vi "Main.vi"(8 "error in":errorcluster, 11 "Server Client in":refnum<class "Server Client.lvclass">) -> (0 "error out":errorcluster, 3 "Server Client out":refnum<class "Server Client.lvclass">)   [LabVIEW 2020, in "Server Client.lvclass"]
doc: "The Queued Message Handler of a Worker."
uses:
  Server Client.lvclass
  <vilib>/addons/_Workers/Library/Classes/EHL/EHL.lvclass
  <vilib>/addons/_Workers/Library/Classes/Worker/Worker.lvclass
  <vilib>/addons/_Workers/Library/Classes/Error Handler/Error Handler.lvclass
  Initialization Data.ctl
  Listener/Listener.lvclass
  <vilib>/addons/_Workers/Library/Classes/Message/Message.lvclass
  <vilib>/addons/_Workers/Library/Classes/Message/Enqueue Message to Queue.vi
  Network End Point/Network End Point.lvclass
  Network End Point/Initialization Data.ctl
  <vilib>/addons/_Workers/Library/Classes/Message Queue/Message Queue.lvclass
  <vilib>/addons/_Workers/Library/Classes/Message/Enqueue Message to Self.vi
  C:/Program Files (x86)/National Instruments/LabVIEW 2020/vi.lib/addons/_Workers/Library/Classes/Worker User/Worker User.lvclass
  C:/Program Files (x86)/National Instruments/LabVIEW 2020/vi.lib/addons/_Workers/Library/Classes/Worker/Worker.lvclass
  C:/Program Files (x86)/National Instruments/LabVIEW 2020/vi.lib/addons/_Workers/Library/Classes/Workers Object/Workers Object.lvclass
  C:/Users/TestAdmin/git/TCP-Workers/Workers/Server Client/Server Client.lvclass
  C:/Users/TestAdmin/git/TCP-Workers/Workers/Listener/Listener.lvclass
  C:/Program Files (x86)/National Instruments/LabVIEW 2020/vi.lib/addons/_Workers/Library/Classes/Message Queue/Message Queue.lvclass
  C:/Users/TestAdmin/git/TCP-Workers/Workers/Network End Point/Network End Point.lvclass
panel:
  in  "Connect to":string
  in  "Open":bool
  in  "Open Listener":bool
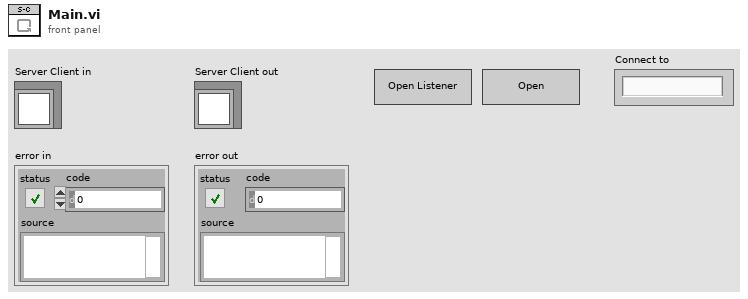
[diagram p1: front panel]
types:
  T1 = typedef "Server Client.lvclass/Initialization Data.ctl" = cluster{"String":string, "port":u16}
  T2 = typedef "Network End Point.lvclass/Initialization Data.ctl" = cluster{"String":string, "Client":string, "connection ID":refnum<k5>, "Caller":refnum<class "Message Queue.lvclass">}
  T3 = typedef "Workers.lvlib/Case Label.ctl" = string
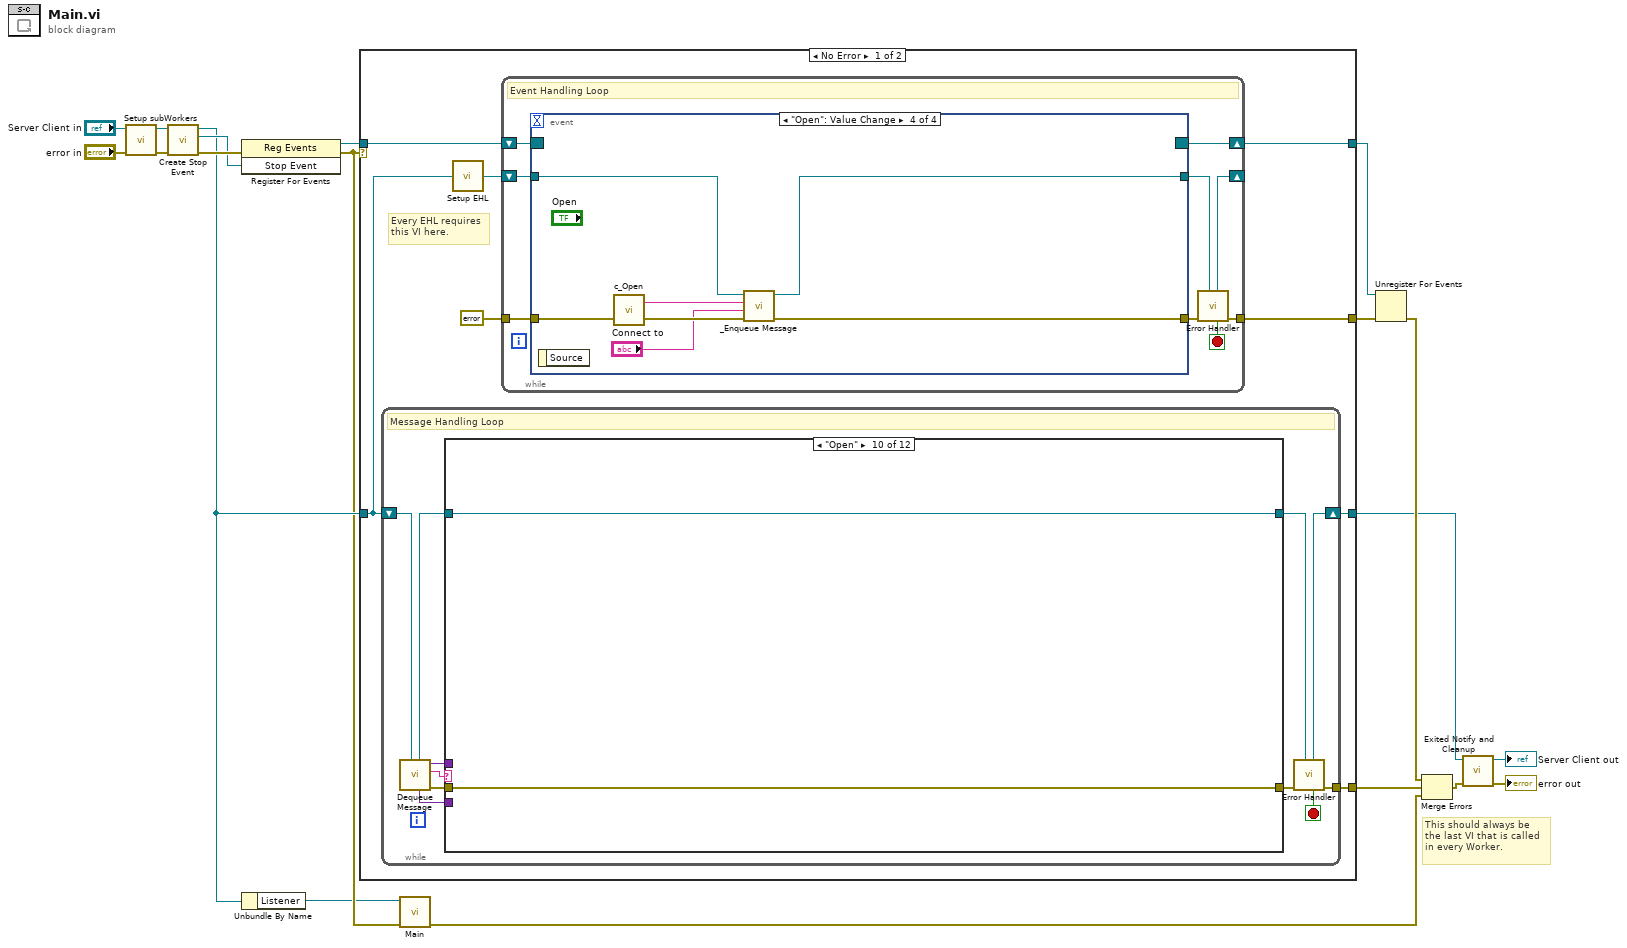
[diagram p0: block diagram]
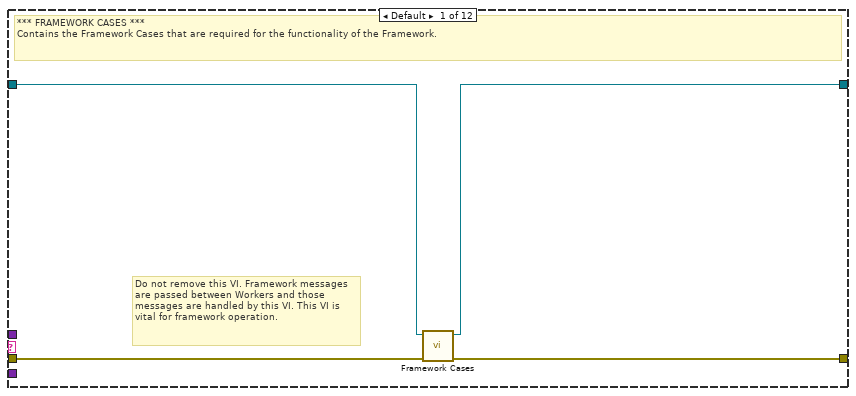
[diagram p2: hidden frame]
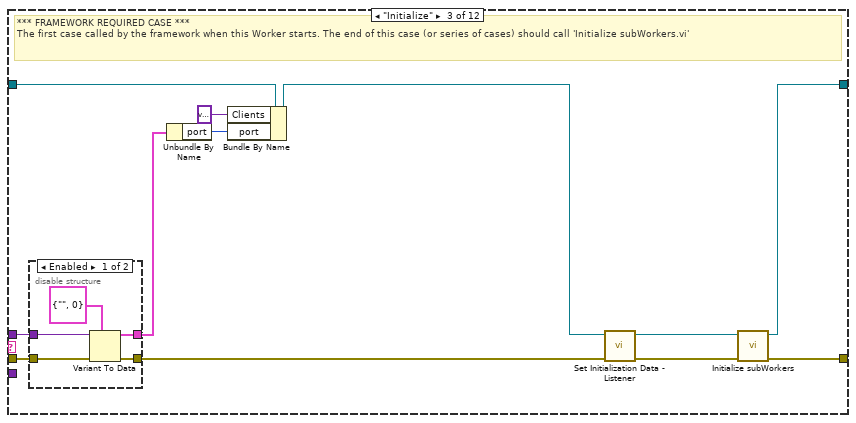
[diagram p4: hidden frame]
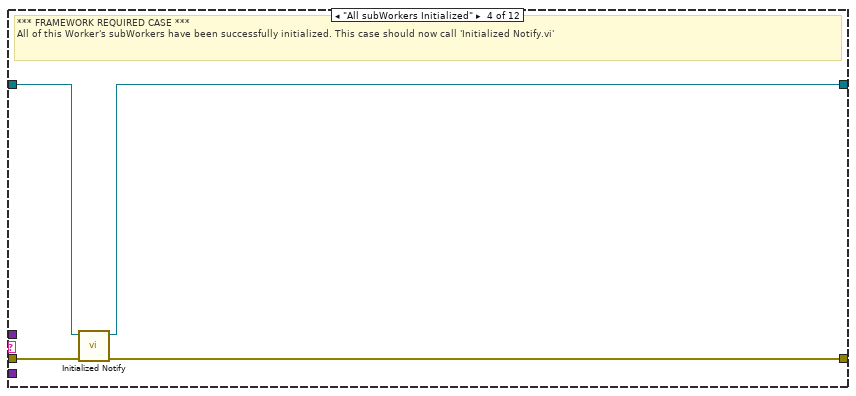
[diagram p6: hidden frame]
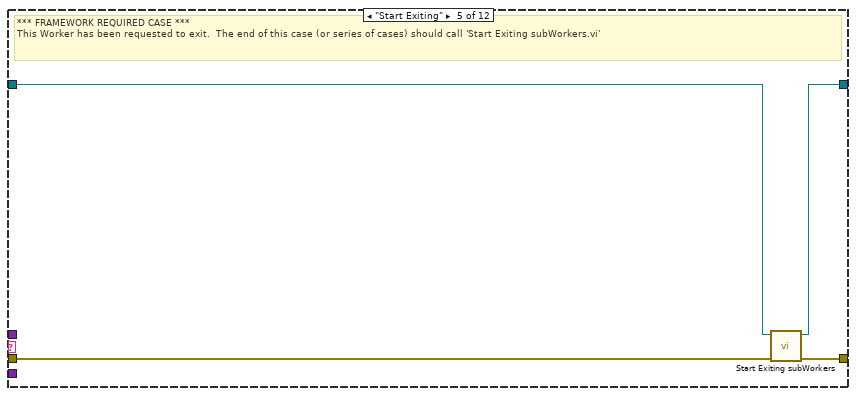
[diagram p7: hidden frame]
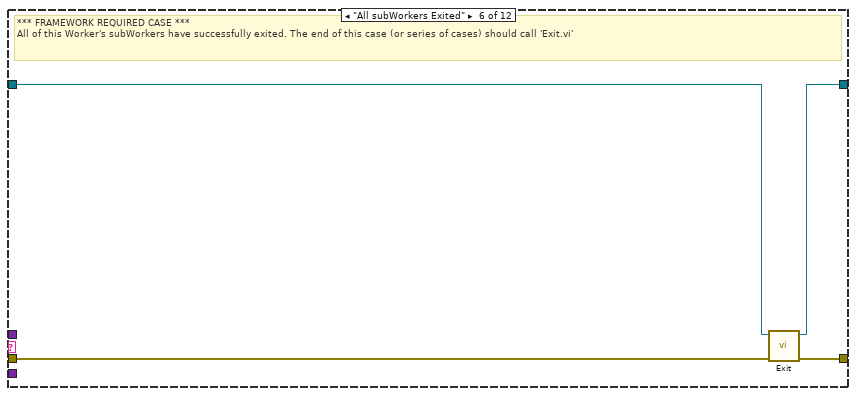
[diagram p8: hidden frame]
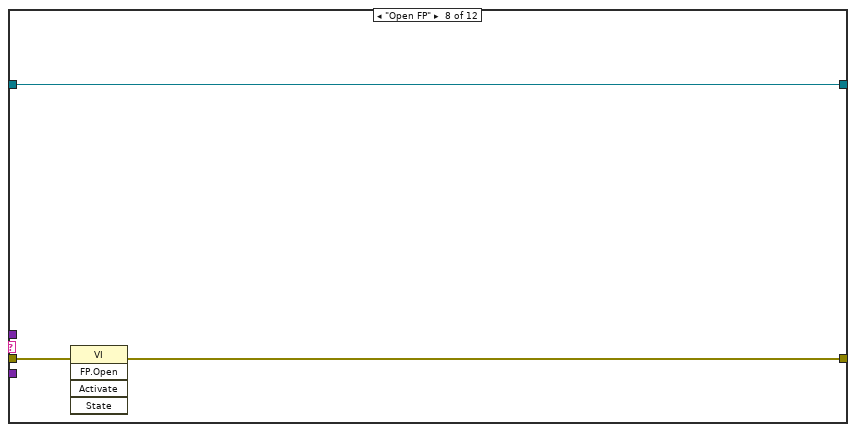
[diagram p10: hidden frame]
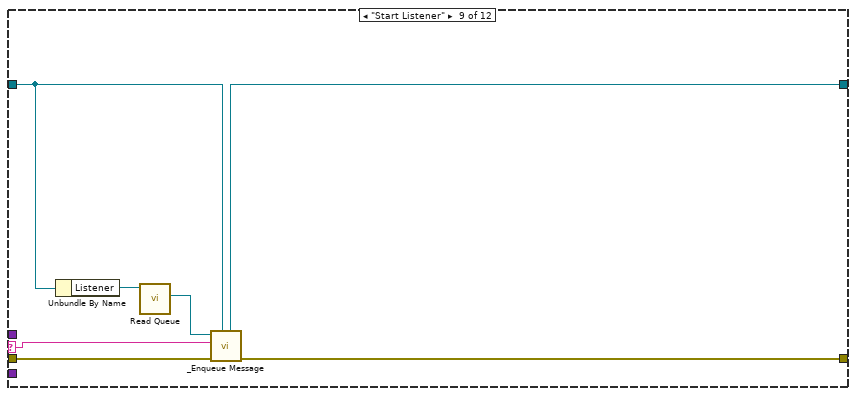
[diagram p11: hidden frame]
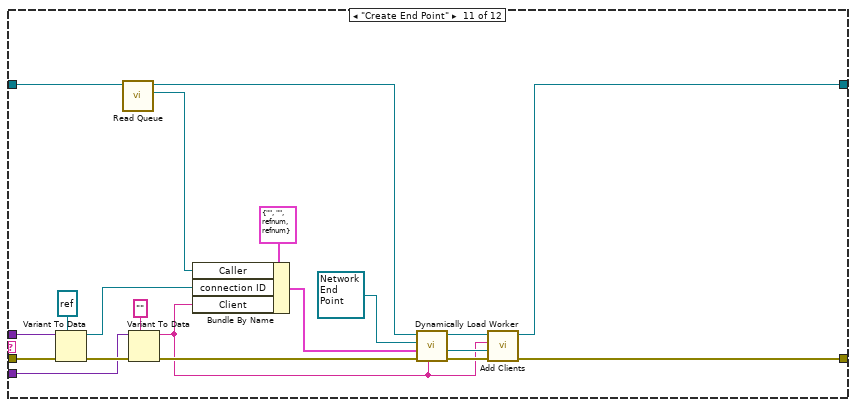
[diagram p12: hidden frame]
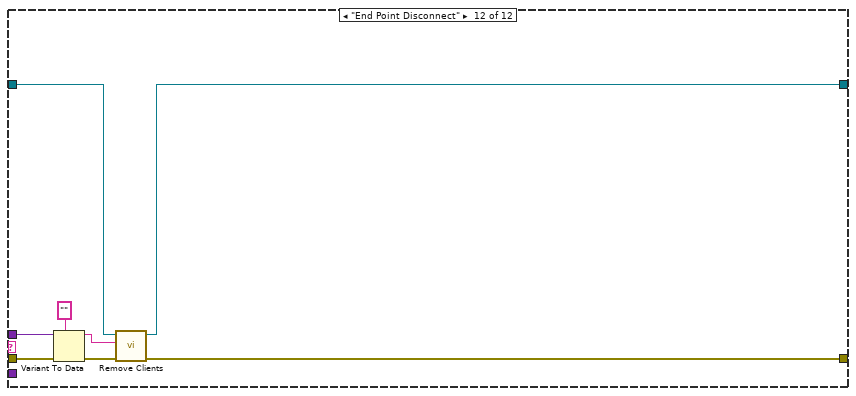
[diagram p13: hidden frame]
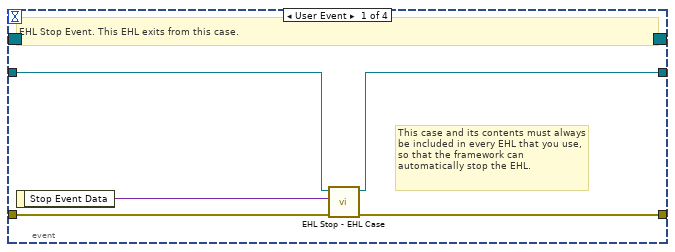
[diagram p14: hidden frame]
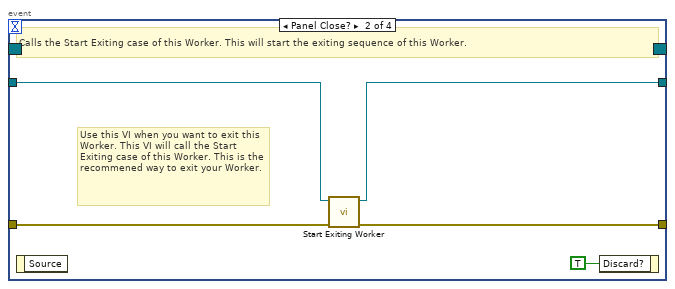
[diagram p15: hidden frame]
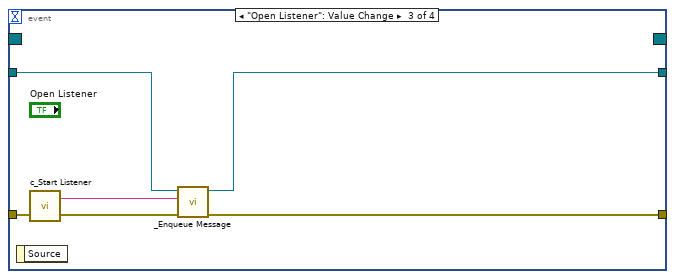
[diagram p16: hidden frame]
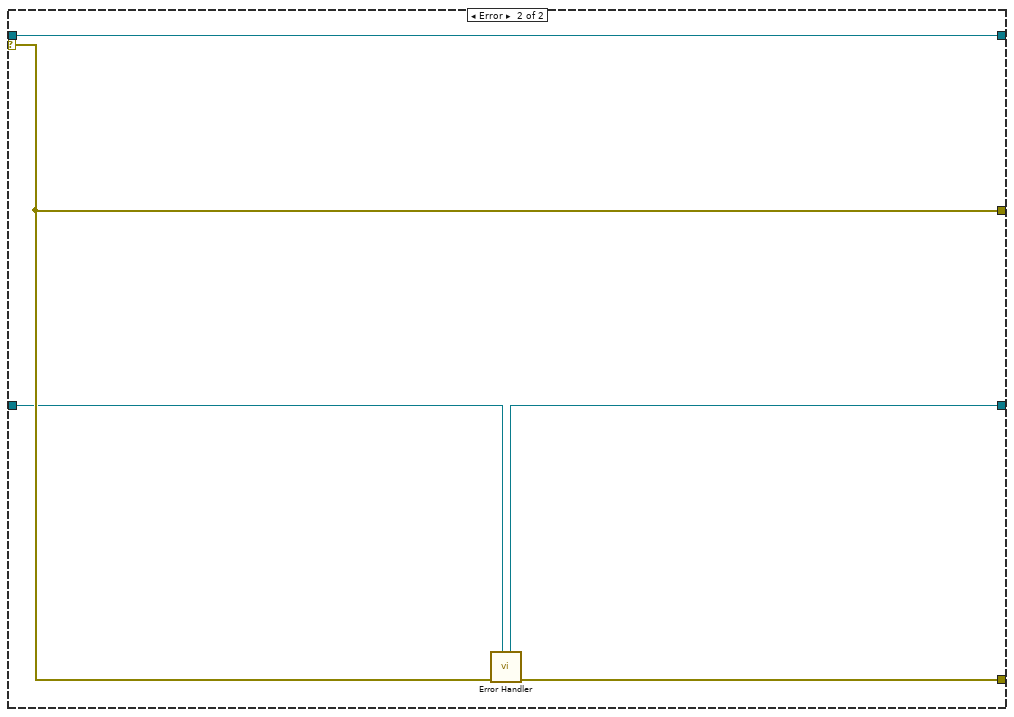
[diagram p17: hidden frame]
diagram:
  # "This should always be the last VI that is called in every Worker."
  n1 = call "Setup subWorkers.vi"("error in"="error in", "Server Client in"="Server Client in") -> ("error out"=w5:errorcluster, "Server Client out"=w3:refnum<class "Server Client.lvclass">)  [unwired: 8 in]
  n2 = call <vilib>:"Create Stop Event.vi"("error in"=w5, "Worker"=w3) -> ("error out"=w14:errorcluster, "Stop Event"=w11:refnum<user-event>, "Worker out"=w8:refnum<class "Server Client.lvclass">)  [unwired: 7 in]
  n3 = register-events(error in=w14, w11) -> (reference out=w13:refnum<event-registration>, error out=w6:errorcluster)  [unwired: 1 in]
  n4 = Unbundle By Name(w8) -> ("Listener"=w2:refnum<class "Listener.lvclass">)
  n5 = case shown="No Error" w6 {
    tunnel: w8 -> [w22 w148]
    tunnel: [w20 w149] -> w12
    tunnel: w13 -> [w27 w150]
    tunnel: [w24 w151] -> w18
    tunnel: [w26 w150] -> w17
    tunnel: [w21 w147] -> w15
    selector: w6 -> [_ w151]
    frame No Error {
      # "Every EHL requires\nthis VI here."
      n6 = while {
        shift-right: [w36] -> w21
        shift-left: w22 -> [w38]
        tunnel: [w37] -> w20
        stop <- w29 stop-if-true
        # "Message Handling Loop"
        n7 = call <vilib>:"Dequeue Message.vi"("Worker"=w38) -> ("error out"=w35:errorcluster, "Case out"=w30:string, "Data out"=w31:variant, "Auxiliary out"=w28:variant, "Worker out"=w33:refnum<class "Server Client.lvclass">)  [unwired: 6 in]
        n8 = case "WORKERS MHL Case Structure (DO NOT CHANGE LABEL NAME)" shown="\"Open\"" w30 {
          selector: w30 -> [_ _ _ _ _ _ _ _ w83 _ _ _]
          tunnel: w35 -> [w42 w43 w54 w66 w67 w74 w75 w79 w86 w87 w108 w116]
          tunnel: [w41 w43 w56 w65 w70 w73 w75 w77 w80 w87 w91 w112] -> w34
          tunnel: w33 -> [w40 w44 w52 w63 w68 w71 w76 w78 w82 w88 w96 w110]
          tunnel: [w39 w44 w55 w64 w69 w72 w76 w78 w81 w88 w93 w109] -> w32
          tunnel: w31 -> [_ _ w53 _ _ _ _ _ _ _ w107 w114]
          tunnel: w28 -> [_ _ _ _ _ _ _ _ _ _ w105 _]
          frame Default {
            # "Do not remove this VI. Framework messages are passed between Workers and those messages are handled by this VI. This VI is vital for framework operation."
            # "*** FRAMEWORK CASES ***\nContains the Framework Cases that are required for the functionality of the Framework."
            n9 = call <vilib>:"Framework Cases.vi"("error in"=w42, "Worker"=w40) -> ("error out"=w41:errorcluster, "Worker out"=w39:refnum<class "Server Client.lvclass">)  [unwired: 8 in]
          }
          frame "------ FRAMEWORK REQUIRED CASES ------" {
            # "Start of Framework Required Cases"
          }
          frame "Initialize" {
            # "*** FRAMEWORK REQUIRED CASE ***\nThe first case called by the framework when this Worker starts. The end of this case (or series of cases) should call 'Initialize subWorkers.vi'"
            n10 = disable-structure shown="Enabled" {
              disable-tunnel: w54 -> [w61 w62]
              disable-tunnel: [w60 w62] -> w49
              disable-tunnel: w53 -> [w59 _]
              disable-tunnel: [w57 _] -> w51
              frame Enabled {
                n11 = Variant To Data(error in=w61, type=T1 {"String"="", "port"=0} ("Initialization Data"), Variant=w59) -> (data=w57:T1, error out=w60:errorcluster)
              }
              frame Disabled {
              }
            }
            n12 = Unbundle By Name(w51) -> ("port"=w50:u16)
            n13 = Bundle By Name(cluster=w52, "Clients"=variant, "port"=w50) -> (w47:refnum<class "Server Client.lvclass">)
            n14 = call "Set Initialization Data - Listener.vi"("error in"=w49, "Server Client in"=w47) -> ("error out"=w48:errorcluster, "Server Client out"=w46:refnum<class "Server Client.lvclass">)  [unwired: 8 in]
            n15 = call <vilib>:"Initialize subWorkers.vi"("error in"=w48, "Worker"=w46) -> ("error out"=w56:errorcluster, "dup Worker out"=w55:refnum<class "Server Client.lvclass">)  [unwired: 8 in]
          }
          frame "All subWorkers Initialized" {
            # "*** FRAMEWORK REQUIRED CASE ***\nAll of this Worker's subWorkers have been successfully initialized. This case should now call 'Initialized Notify.vi'"
            n16 = call <vilib>:"Initialized Notify.vi"("error in"=w66, "Worker"=w63) -> ("error out"=w65:errorcluster, "dup Worker out"=w64:refnum<class "Server Client.lvclass">)  [unwired: 8 in]
          }
          frame "Start Exiting" {
            # "*** FRAMEWORK REQUIRED CASE ***\nThis Worker has been requested to exit.  The end of this case (or series of cases) should call 'Start Exiting subWorkers.vi'"
            n17 = call <vilib>:"Start Exiting subWorkers.vi"("error_in"=w67, "Worker"=w68) -> ("error out"=w70:errorcluster, "dup Worker out"=w69:refnum<class "Server Client.lvclass">)  [unwired: 8 in]
          }
          frame "All subWorkers Exited" {
            # "*** FRAMEWORK REQUIRED CASE ***\nAll of this Worker's subWorkers have successfully exited. The end of this case (or series of cases) should call 'Exit.vi'"
            n18 = call <vilib>:"Exit.vi"("error_in"=w74, "Worker"=w71) -> ("error out"=w73:errorcluster, "dup Worker out"=w72:refnum<class "Server Client.lvclass">)  [unwired: 8 in]
          }
          frame "-----------------------------------------------" {
            # "End of Framework Required Cases"
          }
          frame "Open FP" {
            n19 = invoke class="VI" method="FP.Open"(error in=w79) -> (error out=w77:errorcluster)  [unwired: 4 in, 4 out]
          }
          frame "Start Listener" {
            n20 = Unbundle By Name(w82) -> ("Listener"=w85:refnum<class "Listener.lvclass">)
            n21 = call <vilib>:"Read Queue.vi"("Worker"=w85) -> ("Message Queue out"=w84:refnum<class "Message Queue.lvclass">)  [unwired: 9 in, 1 out]
            n22 = call-poly <vilib>:"_Enqueue Message.vi"("Worker"=w82, "error in"=w86, "Case Label"=w83, "Message Queue"=w84) -> ("error out"=w80:errorcluster, "dup Worker out"=w81:refnum<class "Server Client.lvclass">)  [unwired: 5 in, 1 out]
          }
          frame "Open" {
          }
          frame "Create End Point" {
            n23 = Variant To Data(error in=w108, type=refnum<k5> refnum ("connection ID"), Variant=w107) -> (data=w97:refnum<k5>, error out=w106:errorcluster)
            n24 = call <vilib>:"Read Queue.vi"("Worker"=w96) -> ("Message Queue out"=w94:refnum<class "Message Queue.lvclass">, "dup Worker out"=w95:refnum<class "Server Client.lvclass">)  [unwired: 9 in]
            n25 = Variant To Data(error in=w106, type="", Variant=w105) -> (data=w89:string, error out=w102:errorcluster)
            n26 = Bundle By Name(cluster=T2 {"String"="", "Client"="", "connection ID"=refnum, "Caller"=refnum} ("Initialization Data"), "Caller"=w94, "connection ID"=w97, "Client"=w89) -> (w98:T2)
            n27 = call <vilib>:"Dynamically Load Worker.vi"("Worker Alias"=w89, "error in"=w102, "Initialization Data"=w98, "Worker to Dynamically Load"=refnum<class "Network End Point.lvclass"> refnum ("Network End Point.lvclass"), "Worker"=w95) -> ("error out"=w92:errorcluster, "Message Queue out"=w90:refnum<class "Message Queue.lvclass">, "dup Worker out"=w101:refnum<class "Server Client.lvclass">)  [unwired: 3 in, 1 out]
            n28 = call "Add Clients.vi"("error in (no error)"=w92, "End Point Queue"=w90, "Client"=w89, "Server Client in"=w101) -> ("error out"=w91:errorcluster, "Server Client out"=w93:refnum<class "Server Client.lvclass">)  [unwired: 6 in]
          }
          frame "End Point Disconnect" {
            n29 = Variant To Data(error in=w116, type="", Variant=w114) -> (data=w111:string, error out=w115:errorcluster)
            n30 = call "Remove Clients.vi"("error in (no error)"=w115, "Client"=w111, "Server Client in"=w110) -> ("error out"=w112:errorcluster, "Server Client out"=w109:refnum<class "Server Client.lvclass">)  [unwired: 7 in]
          }
        }
        n31 = call <vilib>:"Error Handler.vi"("Worker"=w32, "error_in"=w34) -> ("error out"=w37:errorcluster, "Stop Loop"=w29:bool, "Worker out"=w36:refnum<class "Server Client.lvclass">)  [unwired: 7 in]
      }
      n32 = call <vilib>:"Setup EHL.vi"("Worker"=w22) -> ("Worker out"=w23:refnum<class "Server Client.lvclass">)  [unwired: 14 in]
      n33 = while "Event Handling Loop" {
        shift-right: [w125] -> w26
        shift-left: w27 -> [w124]
        tunnel: [w120] -> w24
        tunnel: errorcluster {"status"=FALSE, "code"=0, "source"=""} ("error constant") -> [w122]
        shift-right: [w118] -> _
        shift-left: w23 -> [w123]
        stop <- w117 stop-if-true
        # "Event Handling Loop"
        n34 = event shown="[3] \"Open\": Value Change" {
          selector: w124 -> [_ _ _ _]
          dyn-events: [_ _ _ _] -> w125
          timeout: _ -> [_ _ _ _]
          tunnel: [w129 w134 w139 w145] -> w121
          tunnel: w122 -> [w130 w133 w140 w146]
          tunnel: w123 -> [w128 w132 w138 w144]
          tunnel: [w127 w131 w137 w143] -> w119
          event User Event {
            # "This case and its contents must always be included in every EHL that you use, so that the framework can automatically stop the EHL."
            # "EHL Stop Event. This EHL exits from this case."
            n35 = event-data() -> ("Stop Event Data"=w126:variant)  [unwired: 1 in]
            n36 = call <vilib>:"EHL Stop - EHL Case.vi"("error in"=w130, "Stop Event Data"=w126, "Worker"=w128) -> ("error out"=w129:errorcluster, "Worker out"=w127:refnum<class "Server Client.lvclass">)  [unwired: 7 in]
          }
          event Panel Close? {
            # "Use this VI when you want to exit this Worker. This VI will call the Start Exiting case of this Worker. This is the recommened way to exit your Worker."
            # "Calls the Start Exiting case of this Worker. This will start the exiting sequence of this Worker."
            n37 = event-data() -> ()  [unwired: 1 in, 1 out]
            n38 = call <vilib>:"Start Exiting Worker.vi"("error in"=w133, "Worker"=w132) -> ("error out"=w134:errorcluster, "dup Worker out"=w131:refnum<class "Server Client.lvclass">)  [unwired: 8 in]
            n39 = event-data ("Event Filter Node")("Discard?"=TRUE) -> ()  [unwired: 1 in, 1 out]
          }
          event "Open Listener": Value Change {
            n40 = event-data() -> ()  [unwired: 1 in, 1 out]
            n41 = call "c_Start Listener.vi"() -> ("Case Label"=w136:T3)  [unwired: 1 in]
            n42 = call-poly <vilib>:"_Enqueue Message.vi"("error in"=w140, "Case Label"=w136, "Worker"=w138) -> ("error out"=w139:errorcluster, "dup Worker out"=w137:refnum<class "Server Client.lvclass">)  [unwired: 7 in]
          }
          event "Open": Value Change {
            n43 = event-data() -> ()  [unwired: 1 in, 1 out]
            n44 = call "c_Open.vi"() -> ("Case Label"=w142:T3)  [unwired: 1 in]
            n45 = call-poly <vilib>:"_Enqueue Message.vi"("error in"=w146, "Data"="Connect to", "Case Label"=w142, "Worker"=w144) -> ("error out"=w145:errorcluster, "dup Worker out"=w143:refnum<class "Server Client.lvclass">)  [unwired: 6 in]
          }
        }
        n46 = call <vilib>:"Error Handler.vi"("Worker"=w119, "error_in"=w121) -> ("error out"=w120:errorcluster, "Stop Loop"=w117:bool, "Worker out"=w118:refnum<class "Server Client.lvclass">)  [unwired: 7 in]
      }
    }
    frame Error {
      n47 = call <vilib>:"Error Handler.vi"("Worker"=w148, "error_in"=w151) -> ("error out"=w149:errorcluster, "Worker out"=w147:refnum<class "Server Client.lvclass">)  [unwired: 7 in, 1 out]
    }
  }
  n48 = call-dynamic "Main.vi"("error in"=w6, "Listener in"=w2) -> ("error out"=w1:errorcluster)  [unwired: 8 in, 1 out]
  n49 = Unregister For Events(event registration refnum=w17, error in=w18) -> (error out=w19:errorcluster)
  n50 = Merge Errors(w19, w12, w1) -> (w16:errorcluster)
  n51 = call <vilib>:"Exited Notify and Cleanup.vi"("error_in"=w16, "Worker"=w15) -> ("error out"=→"error out":errorcluster, "dup Worker out"=→"Server Client out":refnum<class "Server Client.lvclass">)  [unwired: 8 in]
